vi "Serialize as XML.vi"(8 "error in (no error)":errorcluster, 9 "Nesting Level":i32, 11 "Element in":refnum<class "Element.lvclass">) -> (0 "error out":errorcluster, 2 "XML Fragment":string, 3 "Element out":refnum<class "Element.lvclass">)   [LabVIEW 2026, in "VILab.lvlib" / "Element.lvclass"]
uses:
  Element.lvclass
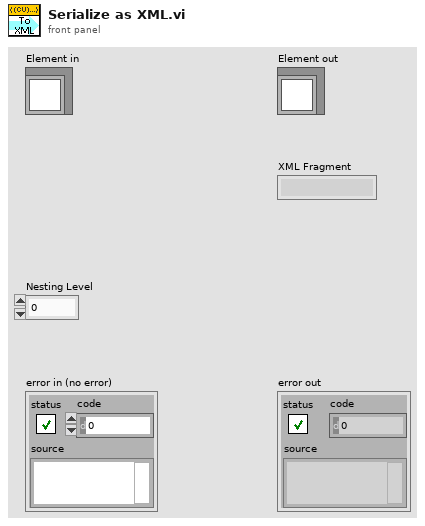
[diagram p1: front panel]
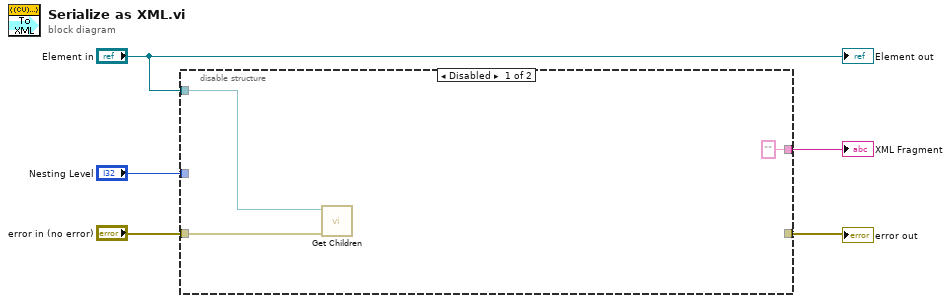
[diagram p0: block diagram]
diagram:
  n1 = disable-structure shown="Disabled" {
    disable-tunnel: "error in (no error)" -> [w8 w9]
    disable-tunnel: [_ w9] -> w4
    disable-tunnel: ["" ("XML Fragment") _] -> w3
    disable-tunnel: "Nesting Level" -> [_ _]
    disable-tunnel: "Element in" -> [w7 _]
    frame Disabled {
      n2 = call-dynamic "Get Children.vi"("error in (no error)"=w8, "Element in"=w7) -> ()  [unwired: 6 in, 4 out]
    }
    frame Enabled {
    }
  }
  "error out" <- w4
  "XML Fragment" <- w3
  "Element out" <- "Element in"
